vi "Timebase and Trigger Routing.vi"(7 "Signal Router Action":T1, 8 "error in":errorcluster, 11 "System Type":string) -> (0 "error out":errorcluster)   [LabVIEW 2012]
uses:
  Timebase and Trigger Routing.ctl
  GFG/GFGstringGet.vi
  GFG/GFG library.lvlib
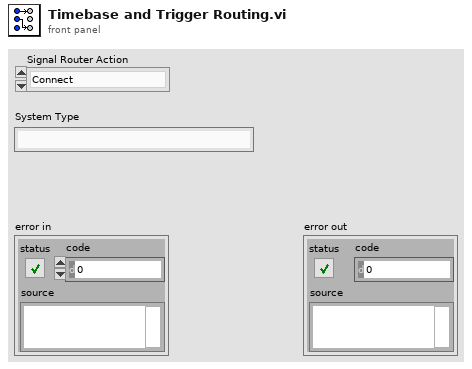
[diagram p1: front panel]
types:
  T1 = typedef "Timebase and Trigger Routing.ctl" = enum16{"Connect", "Disconnect all", "Disconnect Trigger"}
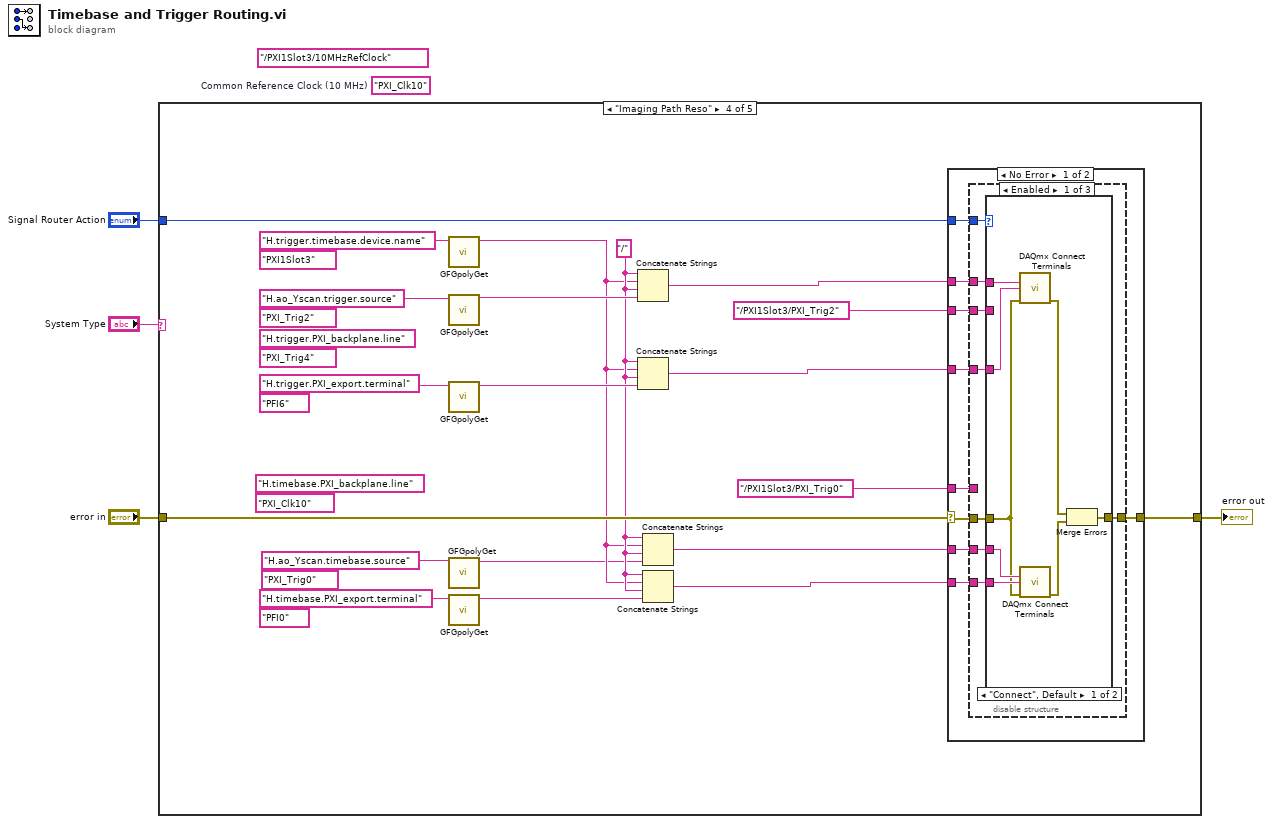
[diagram p0: block diagram]
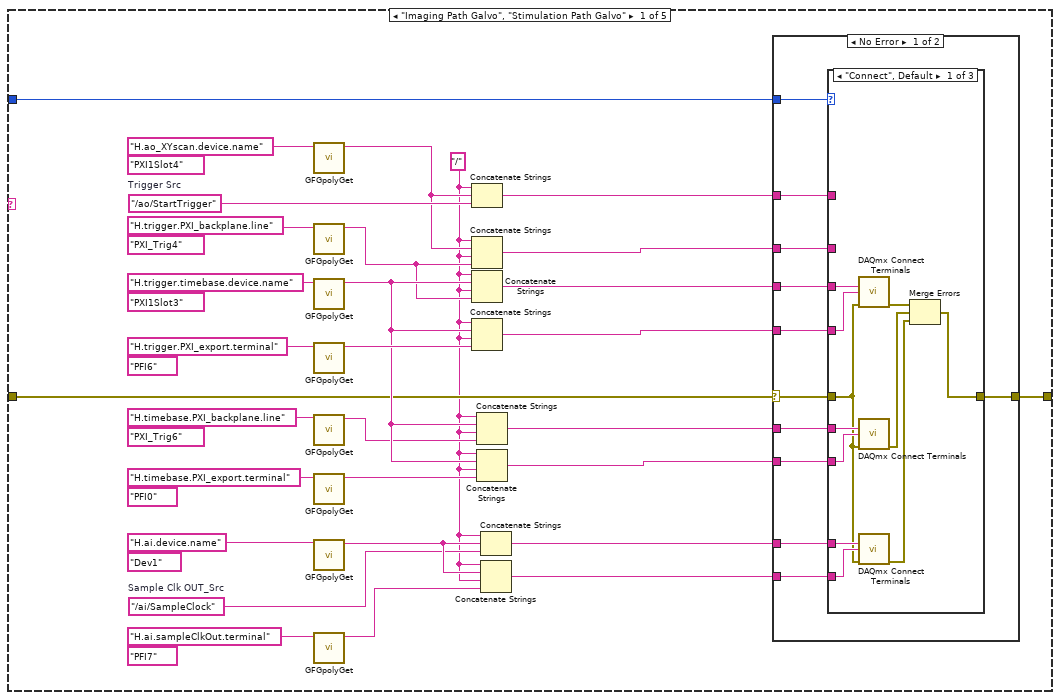
[diagram p2: hidden frame]
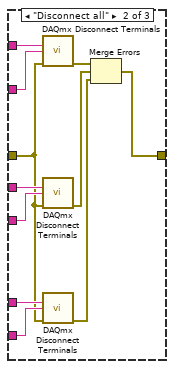
[diagram p3: hidden frame]
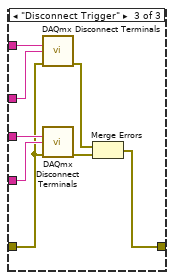
[diagram p4: hidden frame]
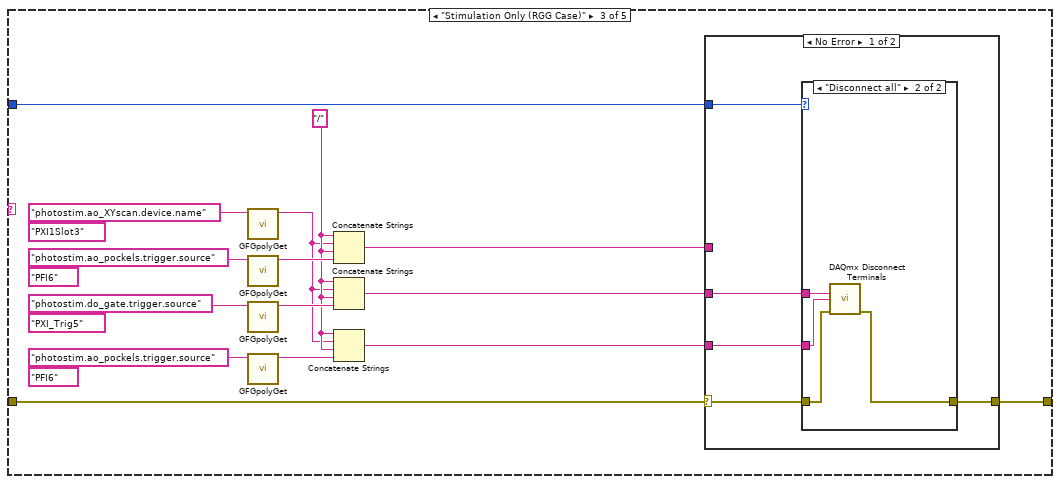
[diagram p7: hidden frame]
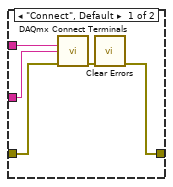
[diagram p8: hidden frame]
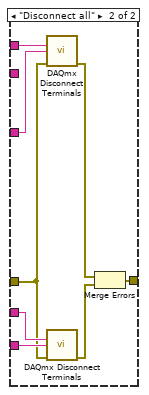
[diagram p10: hidden frame]
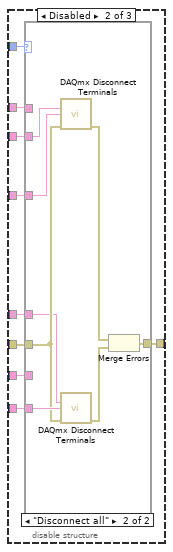
[diagram p11: hidden frame]
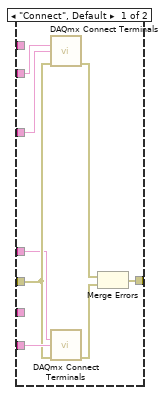
[diagram p12: hidden frame]
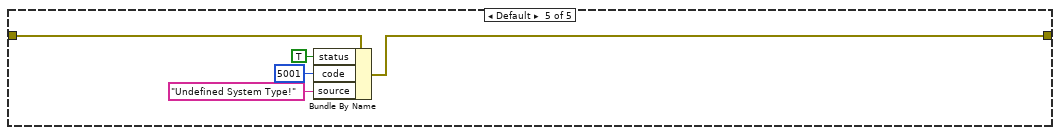
[diagram p15: hidden frame]
diagram:
  (unwired) tag "/PXI1Slot3/10MHzRefClock" ("source terminal")
  (unwired) "PXI_Clk10"  # Common Reference Clock (10 MHz)
  n1 = case shown="\"Imaging Path Reso\"" "System Type" {
    tunnel: [w5 w77 w92 w127 w187] -> w4
    tunnel: "Signal Router Action" -> [w31 _ w91 w126 _]
    tunnel: "error in" -> [w15 w77 w87 w125 w188]
    frame "Imaging Path Galvo", "Stimulation Path Galvo" {
      (unwired) tag "PFI7" ("destination terminal")
      (unwired) tag "Dev1" ("destination terminal")
      (unwired) tag "PXI1Slot4" ("source terminal")
      (unwired) tag "PFI0" ("destination terminal")
      (unwired) tag "PXI_Trig6" ("destination terminal")
      (unwired) tag "PXI1Slot3" ("source terminal")
      (unwired) tag "PFI6" ("destination terminal")
      (unwired) tag "PXI_Trig4" ("source terminal")
      w6 = "/" ("string")
      w27 = "/ai/SampleClock"  # Sample Clk OUT_Src
      w33 = "/ao/StartTrigger"  # Trigger Src
      n2 = call-poly "GFGpolyGet.vi"("Variable Name in"="H.ao_XYscan.device.name" ("AO device name")) -> ("String"=w21:string)  [unwired: 9 in, 1 out]
      n3 = call-poly "GFGpolyGet.vi"("Variable Name in"="H.trigger.PXI_backplane.line") -> ("String"=w9:string)  [unwired: 9 in, 1 out]
      n4 = call-poly "GFGpolyGet.vi"("Variable Name in"="H.trigger.timebase.device.name") -> ("String"=w20:string)  [unwired: 9 in, 1 out]
      n5 = call-poly "GFGpolyGet.vi"("Variable Name in"="H.trigger.PXI_export.terminal") -> ("String"=w34:string)  [unwired: 9 in, 1 out]
      n6 = call-poly "GFGpolyGet.vi"("Variable Name in"="H.timebase.PXI_backplane.line") -> ("String"=w7:string)  [unwired: 9 in, 1 out]
      n7 = call-poly "GFGpolyGet.vi"("Variable Name in"="H.timebase.PXI_export.terminal") -> ("String"=w29:string)  [unwired: 9 in, 1 out]
      n8 = call-poly "GFGpolyGet.vi"("Variable Name in"="H.ai.device.name") -> ("String"=w28:string)  [unwired: 9 in, 1 out]
      n9 = call-poly "GFGpolyGet.vi"("Variable Name in"="H.ai.sampleClkOut.terminal") -> ("String"=w26:string)  [unwired: 9 in, 1 out]
      n10 = Concatenate Strings(w6, w21, w33) -> (w16:string)
      n11 = Concatenate Strings(w6, w21, w6, w9) -> (w17:string)
      n12 = Concatenate Strings(w6, w20, w6, w9) -> (w18:string)
      n13 = Concatenate Strings(w6, w20, w6, w34) -> (w19:string)
      n14 = Concatenate Strings(w6, w20, w6, w7) -> (w14:string)
      n15 = Concatenate Strings(w6, w20, w6, w29) -> (w13:string)
      n16 = Concatenate Strings(w6, w28, w27) -> (w12:string)
      n17 = Concatenate Strings(w6, w28, w6, w26) -> (w11:string)
      n18 = case shown="No Error" w15 {
        selector: w15 -> [w40 w76]
        tunnel: w19 -> [w45 _]
        tunnel: w18 -> [w44 _]
        tunnel: w17 -> [w43 _]
        tunnel: w16 -> [w42 _]
        tunnel: w31 -> [w41 _]
        tunnel: w14 -> [w39 _]
        tunnel: w13 -> [w38 _]
        tunnel: w12 -> [w37 _]
        tunnel: w11 -> [w36 _]
        tunnel: [w35 w76] -> w5
        frame No Error {
          n19 = case shown="\"Connect\", Default" w41 {
            tunnel: w45 -> [w56 w67 w75]
            tunnel: w44 -> [w55 w66 w74]
            tunnel: w43 -> [_ _ w73]
            tunnel: w42 -> [_ _ w72]
            tunnel: w40 -> [w48 w59 w68]
            tunnel: w39 -> [w50 w61 _]
            tunnel: w38 -> [w49 w60 _]
            tunnel: w37 -> [w54 w65 _]
            tunnel: w36 -> [w53 w64 _]
            tunnel: [w52 w63 w69] -> w35
            frame "Connect", Default {
              n20 = call <vilib>:"DAQmx Connect Terminals.vi"("source terminal"=w55, "destination terminal"=w56, "error in"=w48) -> ("error out"=w51:errorcluster)  [unwired: 12 in]
              n21 = call <vilib>:"DAQmx Connect Terminals.vi"("source terminal"=w50, "destination terminal"=w49, "error in"=w48) -> ("error out"=w46:errorcluster)  [unwired: 12 in]
              n22 = call <vilib>:"DAQmx Connect Terminals.vi"("source terminal"=w54, "destination terminal"=w53, "error in"=w48) -> ("error out"=w47:errorcluster)  [unwired: 12 in]
              n23 = Merge Errors(w51, w46, w47) -> (w52:errorcluster)
            }
            frame "Disconnect all" {
              n24 = call <vilib>:"DAQmx Disconnect Terminals.vi"("source terminal"=w66, "destination terminal"=w67, "error in"=w59) -> ("error out"=w62:errorcluster)  [unwired: 12 in]
              n25 = call <vilib>:"DAQmx Disconnect Terminals.vi"("source terminal"=w61, "destination terminal"=w60, "error in"=w59) -> ("error out"=w57:errorcluster)  [unwired: 12 in]
              n26 = call <vilib>:"DAQmx Disconnect Terminals.vi"("source terminal"=w65, "destination terminal"=w64, "error in"=w59) -> ("error out"=w58:errorcluster)  [unwired: 12 in]
              n27 = Merge Errors(w62, w57, w58) -> (w63:errorcluster)
            }
            frame "Disconnect Trigger" {
              n28 = call <vilib>:"DAQmx Disconnect Terminals.vi"("source terminal"=w72, "destination terminal"=w73, "error in"=w68) -> ("error out"=w71:errorcluster)  [unwired: 12 in]
              n29 = call <vilib>:"DAQmx Disconnect Terminals.vi"("source terminal"=w74, "destination terminal"=w75, "error in"=w68) -> ("error out"=w70:errorcluster)  [unwired: 12 in]
              n30 = Merge Errors(w71, w70) -> (w69:errorcluster)
            }
          }
        }
        frame Error {
          # "Undefined system; Don't route!!"
        }
      }
    }
    frame "Stimulation Only (R Path)" {
      # "Nothing happens in routing!"
    }
    frame "Stimulation Only (RGG Case)" {
      (unwired) tag "PFI6" ("source")
      (unwired) tag "PXI_Trig5" ("source")
      (unwired) tag "PFI6" ("source")
      (unwired) tag "PXI1Slot3" ("source")
      w81 = "/" ("string")
      n31 = call-poly "GFGpolyGet.vi"("Variable Name in"="photostim.ao_XYscan.device.name" ("AO device name")) -> ("String"=w80:string)  [unwired: 9 in, 1 out]
      n32 = call-poly "GFGpolyGet.vi"("Variable Name in"="photostim.ao_pockels.trigger.source") -> ("String"=w86:string)  [unwired: 9 in, 1 out]
      n33 = call-poly "GFGpolyGet.vi"("Variable Name in"="photostim.do_gate.trigger.source") -> ("String"=w84:string)  [unwired: 9 in, 1 out]
      n34 = call-poly "GFGpolyGet.vi"("Variable Name in"="photostim.ao_pockels.trigger.source") -> ("String"=w79:string)  [unwired: 9 in, 1 out]
      n35 = Concatenate Strings(w81, w80, w81, w86) -> (w89:string)
      n36 = Concatenate Strings(w81, w80, w81, w84) -> (w83:string)
      n37 = Concatenate Strings(w81, w80, w81, w79) -> (w78:string)
      n38 = case shown="No Error" w87 {
        selector: w87 -> [w95 w107]
        tunnel: w89 -> [_ _]
        tunnel: [w97 w107] -> w92
        tunnel: w91 -> [w96 _]
        tunnel: w83 -> [w94 _]
        tunnel: w78 -> [w93 _]
        frame No Error {
          n39 = case shown="\"Disconnect all\"" w96 {
            tunnel: w93 -> [w102 w106]
            tunnel: w94 -> [w101 w105]
            tunnel: w95 -> [w98 w104]
            tunnel: [w99 w103] -> w97
            frame "Connect", Default {
              n40 = call <vilib>:"DAQmx Connect Terminals.vi"("source terminal"=w101, "destination terminal"=w102, "error in"=w98) -> ("error out"=w100:errorcluster)  [unwired: 12 in]
              n41 = call <vilib>:"Clear Errors.vi"("error in (no error)"=w100) -> ("error out"=w99:errorcluster)  [unwired: 6 in]
            }
            frame "Disconnect all" {
              n42 = call <vilib>:"DAQmx Disconnect Terminals.vi"("source terminal"=w105, "destination terminal"=w106, "error in"=w104) -> ("error out"=w103:errorcluster)  [unwired: 12 in]
            }
          }
        }
        frame Error {
          # "Undefined system; Don't route!!"
        }
      }
    }
    frame "Imaging Path Reso" {
      (unwired) tag "PXI_Clk10" ("source terminal")
      (unwired) "H.timebase.PXI_backplane.line" ("Variable Name in")
      (unwired) tag "PXI_Trig2" ("source terminal")
      (unwired) tag "PFI0" ("source terminal")
      (unwired) tag "PXI_Trig0" ("source terminal")
      (unwired) tag "PXI1Slot3" ("source terminal")
      (unwired) tag "PFI6" ("source terminal")
      (unwired) tag "PXI_Trig4" ("source terminal")
      w116 = "/" ("string")
      (unwired) "H.trigger.PXI_backplane.line" ("Variable Name in")
      n43 = call-poly "GFGpolyGet.vi"("Variable Name in"="H.trigger.timebase.device.name" ("AO device name")) -> ("String"=w115:string)  [unwired: 9 in, 1 out]
      n44 = call-poly "GFGpolyGet.vi"("Variable Name in"="H.ao_Yscan.trigger.source") -> ("String"=w119:string)  [unwired: 9 in, 1 out]
      n45 = call-poly "GFGpolyGet.vi"("Variable Name in"="H.trigger.PXI_export.terminal") -> ("String"=w117:string)  [unwired: 9 in, 1 out]
      n46 = call-poly "GFGpolyGet.vi"("Variable Name in"="H.ao_Yscan.timebase.source") -> ("String"=w114:string)  [unwired: 9 in, 1 out]
      n47 = call-poly "GFGpolyGet.vi"("Variable Name in"="H.timebase.PXI_export.terminal") -> ("String"=w113:string)  [unwired: 9 in, 1 out]
      n48 = Concatenate Strings(w116, w115, w116, w119) -> (w122:string)
      n49 = Concatenate Strings(w116, w115, w116, w117) -> (w123:string)
      n50 = Concatenate Strings(w116, w115, w116, w114) -> (w121:string)
      n51 = Concatenate Strings(w116, w115, w116, w113) -> (w120:string)
      n52 = case shown="No Error" w125 {
        selector: w125 -> [w132 w186]
        tunnel: w123 -> [w136 _]
        tunnel: w122 -> [w135 _]
        tunnel: [w134 w186] -> w127
        tunnel: w126 -> [w133 _]
        tunnel: w121 -> [w131 _]
        tunnel: w120 -> [w130 _]
        tunnel: "/PXI1Slot3/PXI_Trig2" ("Variable Name in") -> [w129 _]
        tunnel: "/PXI1Slot3/PXI_Trig0" ("Variable Name in") -> [w128 _]
        frame No Error {
          n53 = disable-structure shown="Enabled" {
            disable-tunnel: w136 -> [w144 w169 _]
            disable-tunnel: w135 -> [w143 w168 _]
            disable-tunnel: [w142 w167 _] -> w134
            disable-tunnel: w133 -> [w141 w166 _]
            disable-tunnel: w132 -> [w140 w165 _]
            disable-tunnel: w131 -> [w139 w164 _]
            disable-tunnel: w130 -> [w138 w163 _]
            disable-tunnel: w129 -> [w137 w162 _]
            disable-tunnel: w128 -> [_ w161 _]
            frame Enabled {
              n54 = case shown="\"Connect\", Default" w141 {
                tunnel: w144 -> [w152 w160]
                tunnel: w143 -> [w151 w159]
                tunnel: w140 -> [w148 w153]
                tunnel: [w145 w154] -> w142
                tunnel: w139 -> [w150 w158]
                tunnel: w138 -> [w149 w157]
                tunnel: w137 -> [_ _]
                frame "Connect", Default {
                  n55 = call <vilib>:"DAQmx Connect Terminals.vi"("source terminal"=w151, "destination terminal"=w152, "error in"=w148) -> ("error out"=w147:errorcluster)  [unwired: 12 in]
                  n56 = call <vilib>:"DAQmx Connect Terminals.vi"("source terminal"=w150, "destination terminal"=w149, "error in"=w148) -> ("error out"=w146:errorcluster)  [unwired: 12 in]
                  n57 = Merge Errors(w147, w146) -> (w145:errorcluster)
                }
                frame "Disconnect all" {
                  n58 = call <vilib>:"DAQmx Disconnect Terminals.vi"("source terminal"=w159, "destination terminal"=w160, "error in"=w153) -> ("error out"=w156:errorcluster)  [unwired: 12 in]
                  n59 = call <vilib>:"DAQmx Disconnect Terminals.vi"("source terminal"=w158, "destination terminal"=w157, "error in"=w153) -> ("error out"=w155:errorcluster)  [unwired: 12 in]
                  n60 = Merge Errors(w156, w155) -> (w154:errorcluster)
                }
              }
            }
            frame Disabled {
              n61 = case shown="\"Disconnect all\"" w166 {
                tunnel: w169 -> [w177 w185]
                tunnel: w168 -> [_ _]
                tunnel: w165 -> [w175 w180]
                tunnel: [w172 w181] -> w167
                tunnel: w164 -> [_ _]
                tunnel: w163 -> [w176 w184]
                tunnel: w162 -> [w171 w179]
                tunnel: w161 -> [w170 w178]
                frame "Connect", Default {
                  n62 = call <vilib>:"DAQmx Connect Terminals.vi"("source terminal"=w171, "destination terminal"=w177, "error in"=w175) -> ("error out"=w174:errorcluster)  [unwired: 12 in]
                  n63 = call <vilib>:"DAQmx Connect Terminals.vi"("source terminal"=w170, "destination terminal"=w176, "error in"=w175) -> ("error out"=w173:errorcluster)  [unwired: 12 in]
                  n64 = Merge Errors(w174, w173) -> (w172:errorcluster)
                }
                frame "Disconnect all" {
                  n65 = call <vilib>:"DAQmx Disconnect Terminals.vi"("source terminal"=w179, "destination terminal"=w185, "error in"=w180) -> ("error out"=w183:errorcluster)  [unwired: 12 in]
                  n66 = call <vilib>:"DAQmx Disconnect Terminals.vi"("source terminal"=w178, "destination terminal"=w184, "error in"=w180) -> ("error out"=w182:errorcluster)  [unwired: 12 in]
                  n67 = Merge Errors(w183, w182) -> (w181:errorcluster)
                }
              }
            }
            frame Disabled {
            }
          }
        }
        frame Error {
          # "Undefined system; Don't route!!"
        }
      }
    }
    frame Default {
      n68 = Bundle By Name(cluster=w188, "status"=TRUE, "code"=5001, "source"="Undefined System Type!") -> (w187:errorcluster)
    }
  }
  "error out" <- w4
